vi "CFN61G_B87-88-to-Cluster_v1.vi"(11 "Op_Word":u16(slide) scale=0.0..65535.0) -> (3 "output cluster":T1)   [LabVIEW 2017]
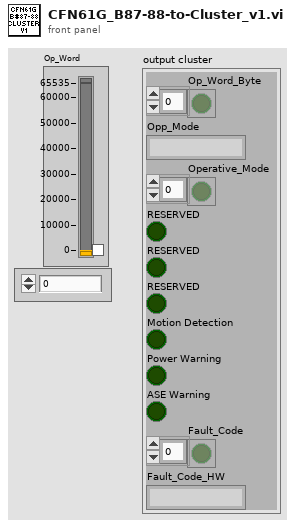
[diagram p1: front panel]
types:
  T1 = cluster{"Op_Word_Byte":bool[], "Opp_Mode":string, "Operative_Mode":bool[], "RESERVED":bool, "RESERVED":bool, "RESERVED":bool, "Motion Detection":bool, "Power Warning":bool, "ASE Warning":bool, "Fault_Code":bool[], "Fault_Code_HW":string}
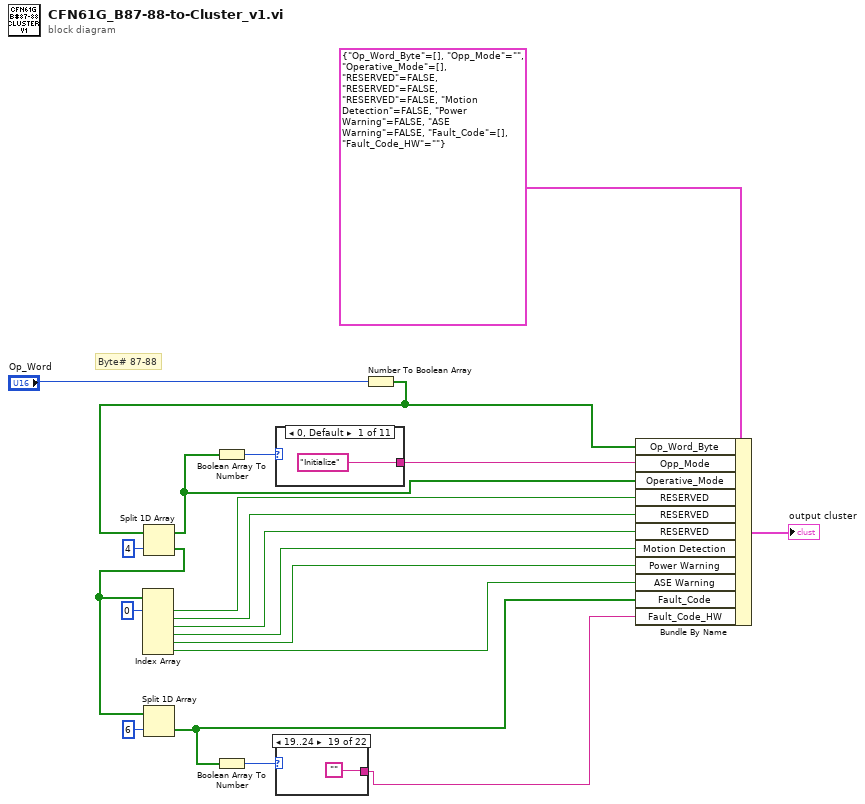
[diagram p0: block diagram]
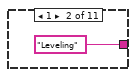
[diagram p2: hidden frame]
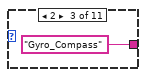
[diagram p3: hidden frame]
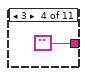
[diagram p4: hidden frame]
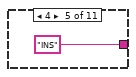
[diagram p5: hidden frame]
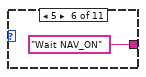
[diagram p6: hidden frame]
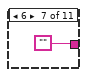
[diagram p7: hidden frame]
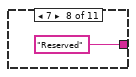
[diagram p8: hidden frame]
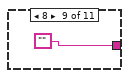
[diagram p9: hidden frame]
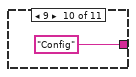
[diagram p10: hidden frame]
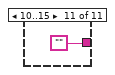
[diagram p11: hidden frame]
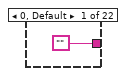
[diagram p12: hidden frame]
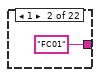
[diagram p13: hidden frame]
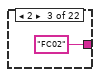
[diagram p14: hidden frame]
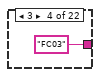
[diagram p15: hidden frame]
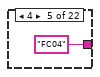
[diagram p16: hidden frame]
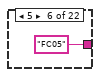
[diagram p17: hidden frame]
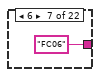
[diagram p18: hidden frame]
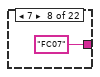
[diagram p19: hidden frame]
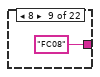
[diagram p20: hidden frame]
diagram:
  # "Byte# 87-88"
  n1 = Number To Boolean Array(number="Op_Word") -> (Boolean array=w18:bool[])
  n2 = Split 1D Array(array=w18, index=4) -> (first subarray=w19:bool[], second subarray=w6:bool[])
  n3 = Index Array(array=w6, index #1=0 ("index")) -> (element #1=w8:bool, element #2=w9:bool, element #3=w10:bool, element #4=w11:bool, element #5=w12:bool, element #6=w13:bool)  [unwired: 5 in]
  n4 = Split 1D Array(array=w6, index=6) -> (second subarray=w14:bool[])  [unwired: 1 out]
  n5 = Boolean Array To Number(Boolean array=w19) -> (number=w5:u32)
  n6 = Boolean Array To Number(Boolean array=w14) -> (number=w4:u32)
  n7 = case shown="0, Default" w5 {
    tunnel: ["Initialize" "Leveling" "Gyro_Compass" "" "INS" "Wait NAV_ON" "" "Reserved" "" "Config" ""] -> w17
    frame 0, Default {
    }
    frame 1 {
    }
    frame 2 {
    }
    frame 3 {
    }
    frame 4 {
    }
    frame 5 {
    }
    frame 6 {
    }
    frame 7 {
    }
    frame 8 {
    }
    frame 9 {
    }
    frame 10..15 {
    }
  }
  n8 = case shown="19..24" w4 {
    tunnel: ["" "FC01" "FC02" "FC03" "FC04" "FC05" "FC06" "FC07" "FC08" "FC09" "" "FC12" "FC13" "FC14" "FC15" "FC16" "FC17" "FC18" "" "FC25" "" "FC36"] -> w15
    frame 0, Default {
    }
    frame 1 {
    }
    frame 2 {
    }
    frame 3 {
    }
    frame 4 {
    }
    frame 5 {
    }
    frame 6 {
    }
    frame 7 {
    }
    frame 8 {
    }
    frame 9 {
    }
    frame 10, 11 {
    }
    frame 12 {
    }
    frame 13 {
    }
    frame 14 {
    }
    frame 15 {
    }
    frame 16 {
    }
    frame 17 {
    }
    frame 18 {
    }
    frame 19..24 {
    }
    frame 25 {
    }
    frame 26..35 {
    }
    frame 36 {
    }
  }
  n9 = Bundle By Name(cluster=T1 {"Op_Word_Byte"=[], "Opp_Mode"="", "Operative_Mode"=[], "RESERVED"=FALSE, "RESERVED"=FALSE, "RESERVED"=FALSE, "Motion Detection"=FALSE, "Power Warning"=FALSE, "ASE Warning"=FALSE, "Fault_Code"=[], "Fault_Code_HW"=""}, "Op_Word_Byte"=w18, "Opp_Mode"=w17, "Operative_Mode"=w19, "RESERVED"=w8, "RESERVED"=w9, "RESERVED"=w10, "Motion Detection"=w11, "Power Warning"=w12, "ASE Warning"=w13, "Fault_Code"=w14, "Fault_Code_HW"=w15) -> (→"output cluster":T1)
